vi "GetConnectionInfo.vi"(7 "LabVIEW Web Service Request":refnum<class "Web Request.lvclass">) -> ()   [LabVIEW 2017]
uses:
  <vilib>/wsapi/Web Request.lvclass
  <vilib>/addons/InsightCM/Devices/Shared/Common/ServerComm/ServerComm.lvlib
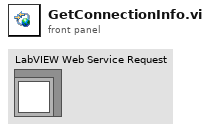
[diagram p1: front panel]
types:
  T1 = typedef "ConnectionInfo.ctl" = cluster{"ClientName":string, "TransceiverHost":string, "TransceiverPort":u16, "Password":string}
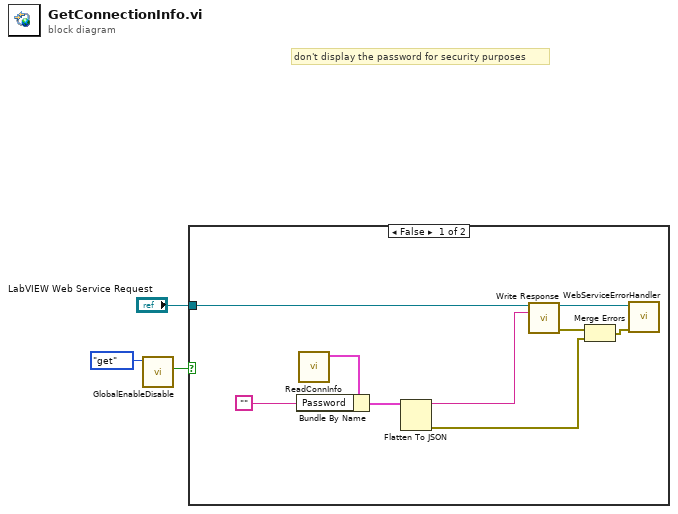
[diagram p0: block diagram]
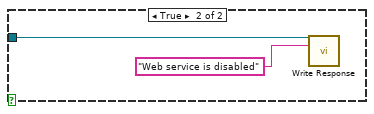
[diagram p2: hidden frame]
diagram:
  # "don't display the password for security purposes"
  n1 = call "GlobalEnableDisable.vi"("action"=enum16{"init", "set", "get"}."get") -> ("DisableDeviceWebService"=w1:bool)  [unwired: 10 in]
  n2 = case shown="False" w1 {
    tunnel: "LabVIEW Web Service Request" -> [w12 w13]
    frame False {
      n3 = call <vilib>:"ReadConnInfo.vi"() -> ("connection info"=w6:T1)  [unwired: 9 in, 2 out]
      n4 = Bundle By Name(cluster=w6, "Password"="") -> (w8:T1)
      n5 = Flatten To JSON(anything=w8) -> (JSON string=w11:string, 11:w4:errorcluster)  [unwired: 2 in]
      n6 = call <vilib>:"Write Response.vi"("LabVIEW Web Service Request"=w12, "response string"=w11) -> ("LabVIEW Web Service Request out"=w10:refnum<class "Web Request.lvclass">, "error out"=w9:errorcluster)  [unwired: 12 in]
      n7 = Merge Errors(w9, w4) -> (w5:errorcluster)
      n8 = call "WebServiceErrorHandler.vi"("LabVIEW Web Service Request"=w10, "error in (no error)"=w5) -> ()  [unwired: 12 in, 2 out]
    }
    frame True {
      n9 = call <vilib>:"Write Response.vi"("LabVIEW Web Service Request"=w13, "response string"="Web service is disabled") -> ()  [unwired: 12 in, 2 out]
    }
  }
